vi "Write Sync Mode.vi"(8 "error in (no error)":errorcluster, 11 "Application in":refnum<class "Application.lvclass">) -> (0 "error out":errorcluster, 3 "Application out":refnum<class "Application.lvclass">)   [LabVIEW 2018, in "Application.lvclass"]
doc: "Este VI apresenta uma interface para que o usuário escolha o modo de sincronização das câmeras."
uses:
  Application.lvclass
  Application.lvclass/Application.ctl
panel:
  in  "OK Button":bool
  in  "Sync Mode:":T1(radio)
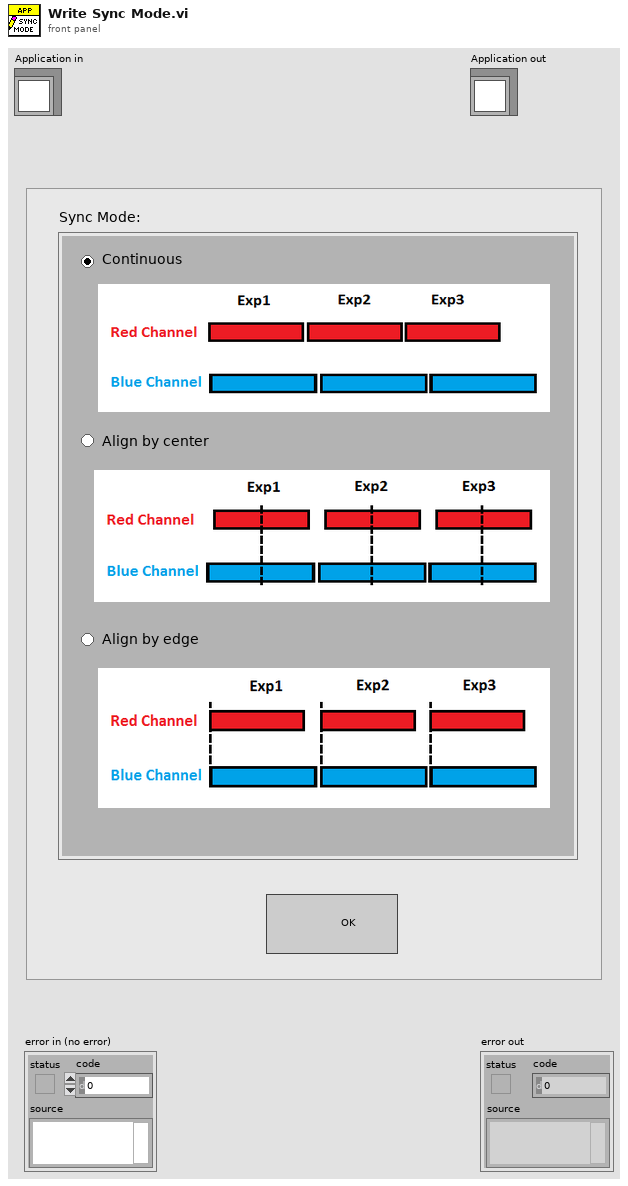
[diagram p1: front panel]
types:
  T1 = enum32{"Radio Selection 1", "Radio Selection 2", "Radio Selection 3"}
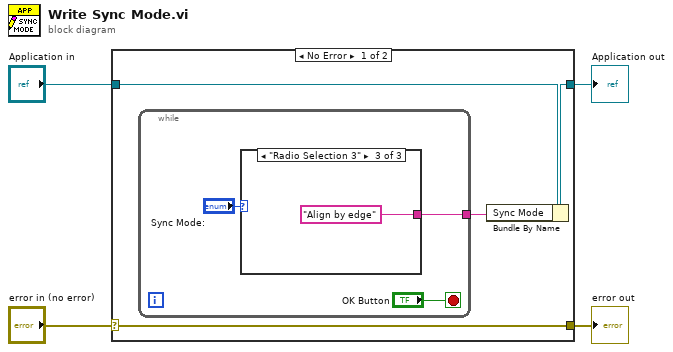
[diagram p0: block diagram]
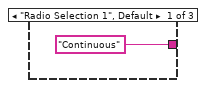
[diagram p2: hidden frame]
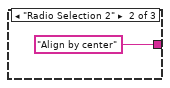
[diagram p3: hidden frame]
diagram:
  n1 = case shown="No Error" "error in (no error)" {
    selector: "error in (no error)" -> [w8 w15]
    tunnel: [w8 w15] -> w3
    tunnel: [w6 w16] -> w1
    tunnel: "Application in" -> [w7 w16]
    frame No Error {
      n2 = while {
        tunnel: [w10] -> w5
        stop <- "OK Button" stop-if-true
        n3 = case shown="\"Radio Selection 3\"" "Sync Mode:" {
          tunnel: ["Continuous" "Align by center" "Align by edge"] -> w10
          frame "Radio Selection 1", Default {
          }
          frame "Radio Selection 2" {
          }
          frame "Radio Selection 3" {
          }
        }
      }
      n4 = Bundle By Name(cluster=w7, "Sync Mode"=w5) -> (w6:refnum<class "Application.lvclass">)
    }
    frame Error {
    }
  }
  "error out" <- w3
  "Application out" <- w1
